vi "Save data file (stop) v3.vi"(11 "panel id":string) -> (0 "network file save error":errorcluster, 3 "file save path":string)   [LabVIEW 2017]
uses:
  Global 1.vi
panel:
  out "C drive root path":string
  out "network file dir path":path
  out "network dir":string
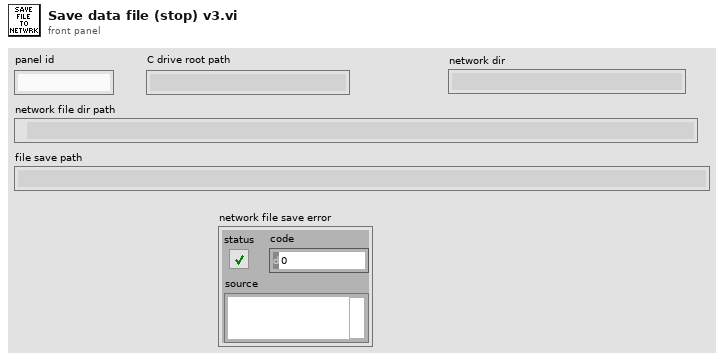
[diagram p1: front panel]
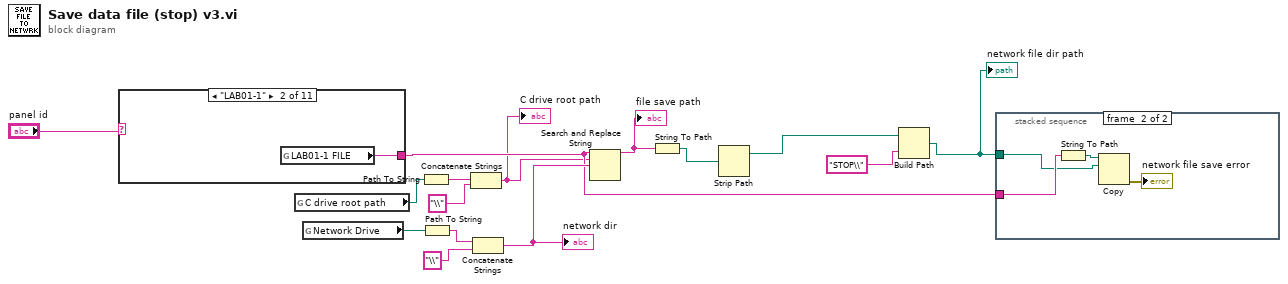
[diagram p0: block diagram]
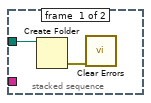
[diagram p2: hidden frame]
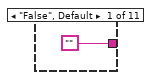
[diagram p3: hidden frame]
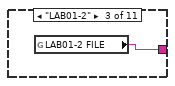
[diagram p4: hidden frame]
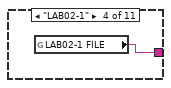
[diagram p5: hidden frame]
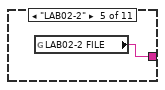
[diagram p6: hidden frame]
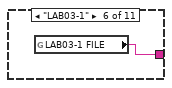
[diagram p7: hidden frame]
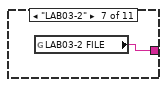
[diagram p8: hidden frame]
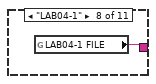
[diagram p9: hidden frame]
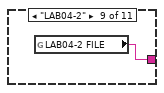
[diagram p10: hidden frame]
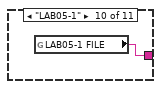
[diagram p11: hidden frame]
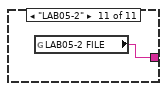
[diagram p12: hidden frame]
diagram:
  n1 = case shown="\"LAB01-1\"" "panel id" {
    tunnel: ["" w17 w18 w19 w20 w21 w22 w23 w24 w25 w26] -> w8
    frame "False", Default {
    }
    frame "LAB01-1" {
      n2 = global read "Global 1.vi" "LAB01-1 FILE"() -> (w17:string)
    }
    frame "LAB01-2" {
      n3 = global read "Global 1.vi" "LAB01-2 FILE"() -> (w18:string)
    }
    frame "LAB02-1" {
      n4 = global read "Global 1.vi" "LAB02-1 FILE"() -> (w19:string)
    }
    frame "LAB02-2" {
      n5 = global read "Global 1.vi" "LAB02-2 FILE"() -> (w20:string)
    }
    frame "LAB03-1" {
      n6 = global read "Global 1.vi" "LAB03-1 FILE"() -> (w21:string)
    }
    frame "LAB03-2" {
      n7 = global read "Global 1.vi" "LAB03-2 FILE"() -> (w22:string)
    }
    frame "LAB04-1" {
      n8 = global read "Global 1.vi" "LAB04-1 FILE"() -> (w23:string)
    }
    frame "LAB04-2" {
      n9 = global read "Global 1.vi" "LAB04-2 FILE"() -> (w24:string)
    }
    frame "LAB05-1" {
      n10 = global read "Global 1.vi" "LAB05-1 FILE"() -> (w25:string)
    }
    frame "LAB05-2" {
      n11 = global read "Global 1.vi" "LAB05-2 FILE"() -> (w26:string)
    }
  }
  n12 = global read "Global 1.vi" "C drive root path"() -> (w5:path)
  n13 = global read "Global 1.vi" "Network Drive"() -> (w14:path)
  n14 = Path To String(path=w5) -> (string=w6:string)
  n15 = Path To String(path=w14) -> (string=w13:string)
  n16 = Concatenate Strings(w6, "\\") -> (w4:string)
  "C drive root path" <- w4
  n17 = Concatenate Strings(w13, "\\") -> (w11:string)
  "network dir" <- w11
  n18 = Search and Replace String(input string=w8, search string=w4, replace string=w11) -> (result string=w10:string)  [unwired: 5 in, 3 out]
  "file save path" <- w10
  n19 = String To Path(string=w10) -> (path=w9:path)
  n20 = Strip Path(path=w9) -> (stripped path=w2:path)  [unwired: 1 out]
  n21 = Build Path(base path=w2, name or relative path="STOP\\") -> (appended path=w1:path)
  "network file dir path" <- w1
  n22 = stacked-sequence {
    tunnel: w1 -> [w28 w29]
    tunnel: w8 -> [_ w30]
    frame #0 {
      n23 = Create Folder(path (use dialog)=w28) -> (error out=w27:errorcluster)  [unwired: 2 in, 2 out]
      n24 = call <vilib>:"Clear Errors.vi"("error in (no error)"=w27) -> ()  [unwired: 5 in, 2 out]
    }
    frame #1 {
      n25 = String To Path(string=w30) -> (path=w31:path)
      n26 = Copy(10:w29, 11:w31) -> (0:→"network file save error":errorcluster)  [unwired: 3 in, 2 out]
    }
  }
